vi "Offline_Analysis_SWSVM_newSelectionMethod_in_분석기_woF4.vi"(0 "LDA_matrix":path caption="LDA_matrix.txt", 1 "svm_model_file":string, 3 "Target_order.txt":path, 4 "mius_flash_order":path, 5 "Brain":path, 6 "Target":path, 7 "피험자이름":string="홍길동", 8 "Nontarget":path, 10 "DIscard Channel Info":i32[](array[numeric]), 11 "Save_path":string, 12 "in_matrix":path caption="in") -> ()   [LabVIEW 2014]
uses:
  <vilib>/Utility/file.llb/Read From Spreadsheet File (DBL).vi
  <vilib>/Analysis/Matrix/Numeric/Conversions/Array To Matrix - RA2.vi
  <vilib>/Analysis/Matrix/Numeric/Conversions/Array To Matrix - RA.vi
  <vilib>/Utility/file.llb/Read From Spreadsheet File (I64).vi
  <vilib>/Utility/file.llb/Write To Spreadsheet File (DBL).vi
  <vilib>/Utility/file.llb/Write To Spreadsheet File (I64).vi
  <vilib>/Utility/file.llb/Write To Spreadsheet File (string).vi
  <vilib>/Analysis/Matrix/NI_Matrix.lvlib
panel:
  out "ACC":i16
  out "Target_order":i64[](array[numeric])
  out "Selected_Target":i32[](array[numeric])
  out "Accuracy":i16[](array[numeric])
  out "error out":errorcluster
  in  "Random_num":i32=6
  in  "Flash_Repeat":i32=20
  in  "Frame_Length":i32=10
  in  "Sampling_Rate":dbl=250.0
  # "ERP_Parameter안씀. LDA바로 집어넣으면 됨"
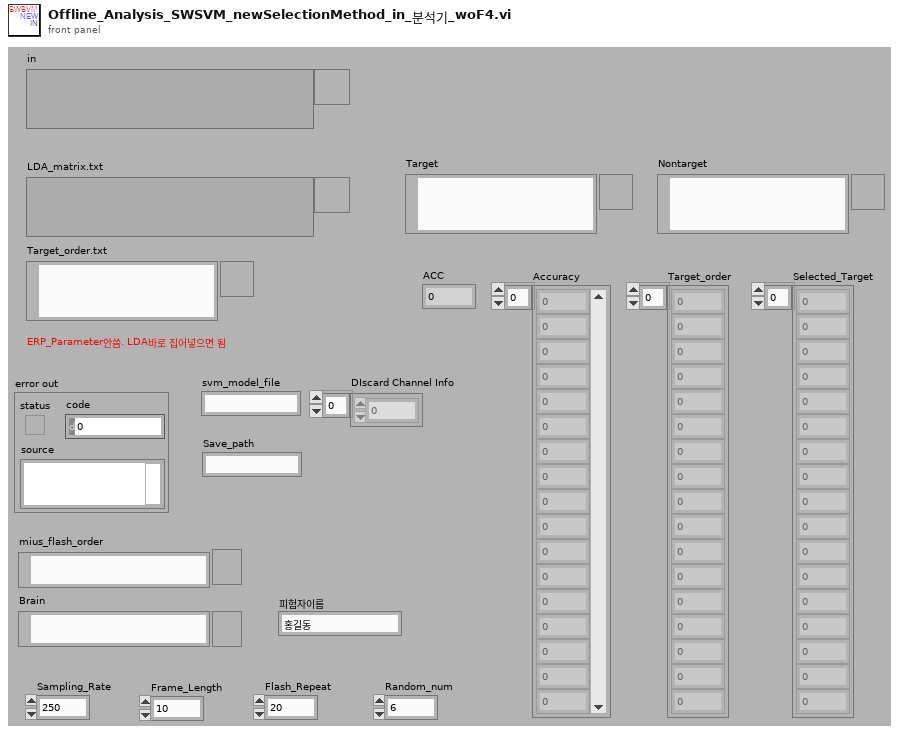
[diagram p1: front panel]
types:
  T1 = typedef "NI_Matrix.lvlib/RealMatrix.ctl" = dbl[][]
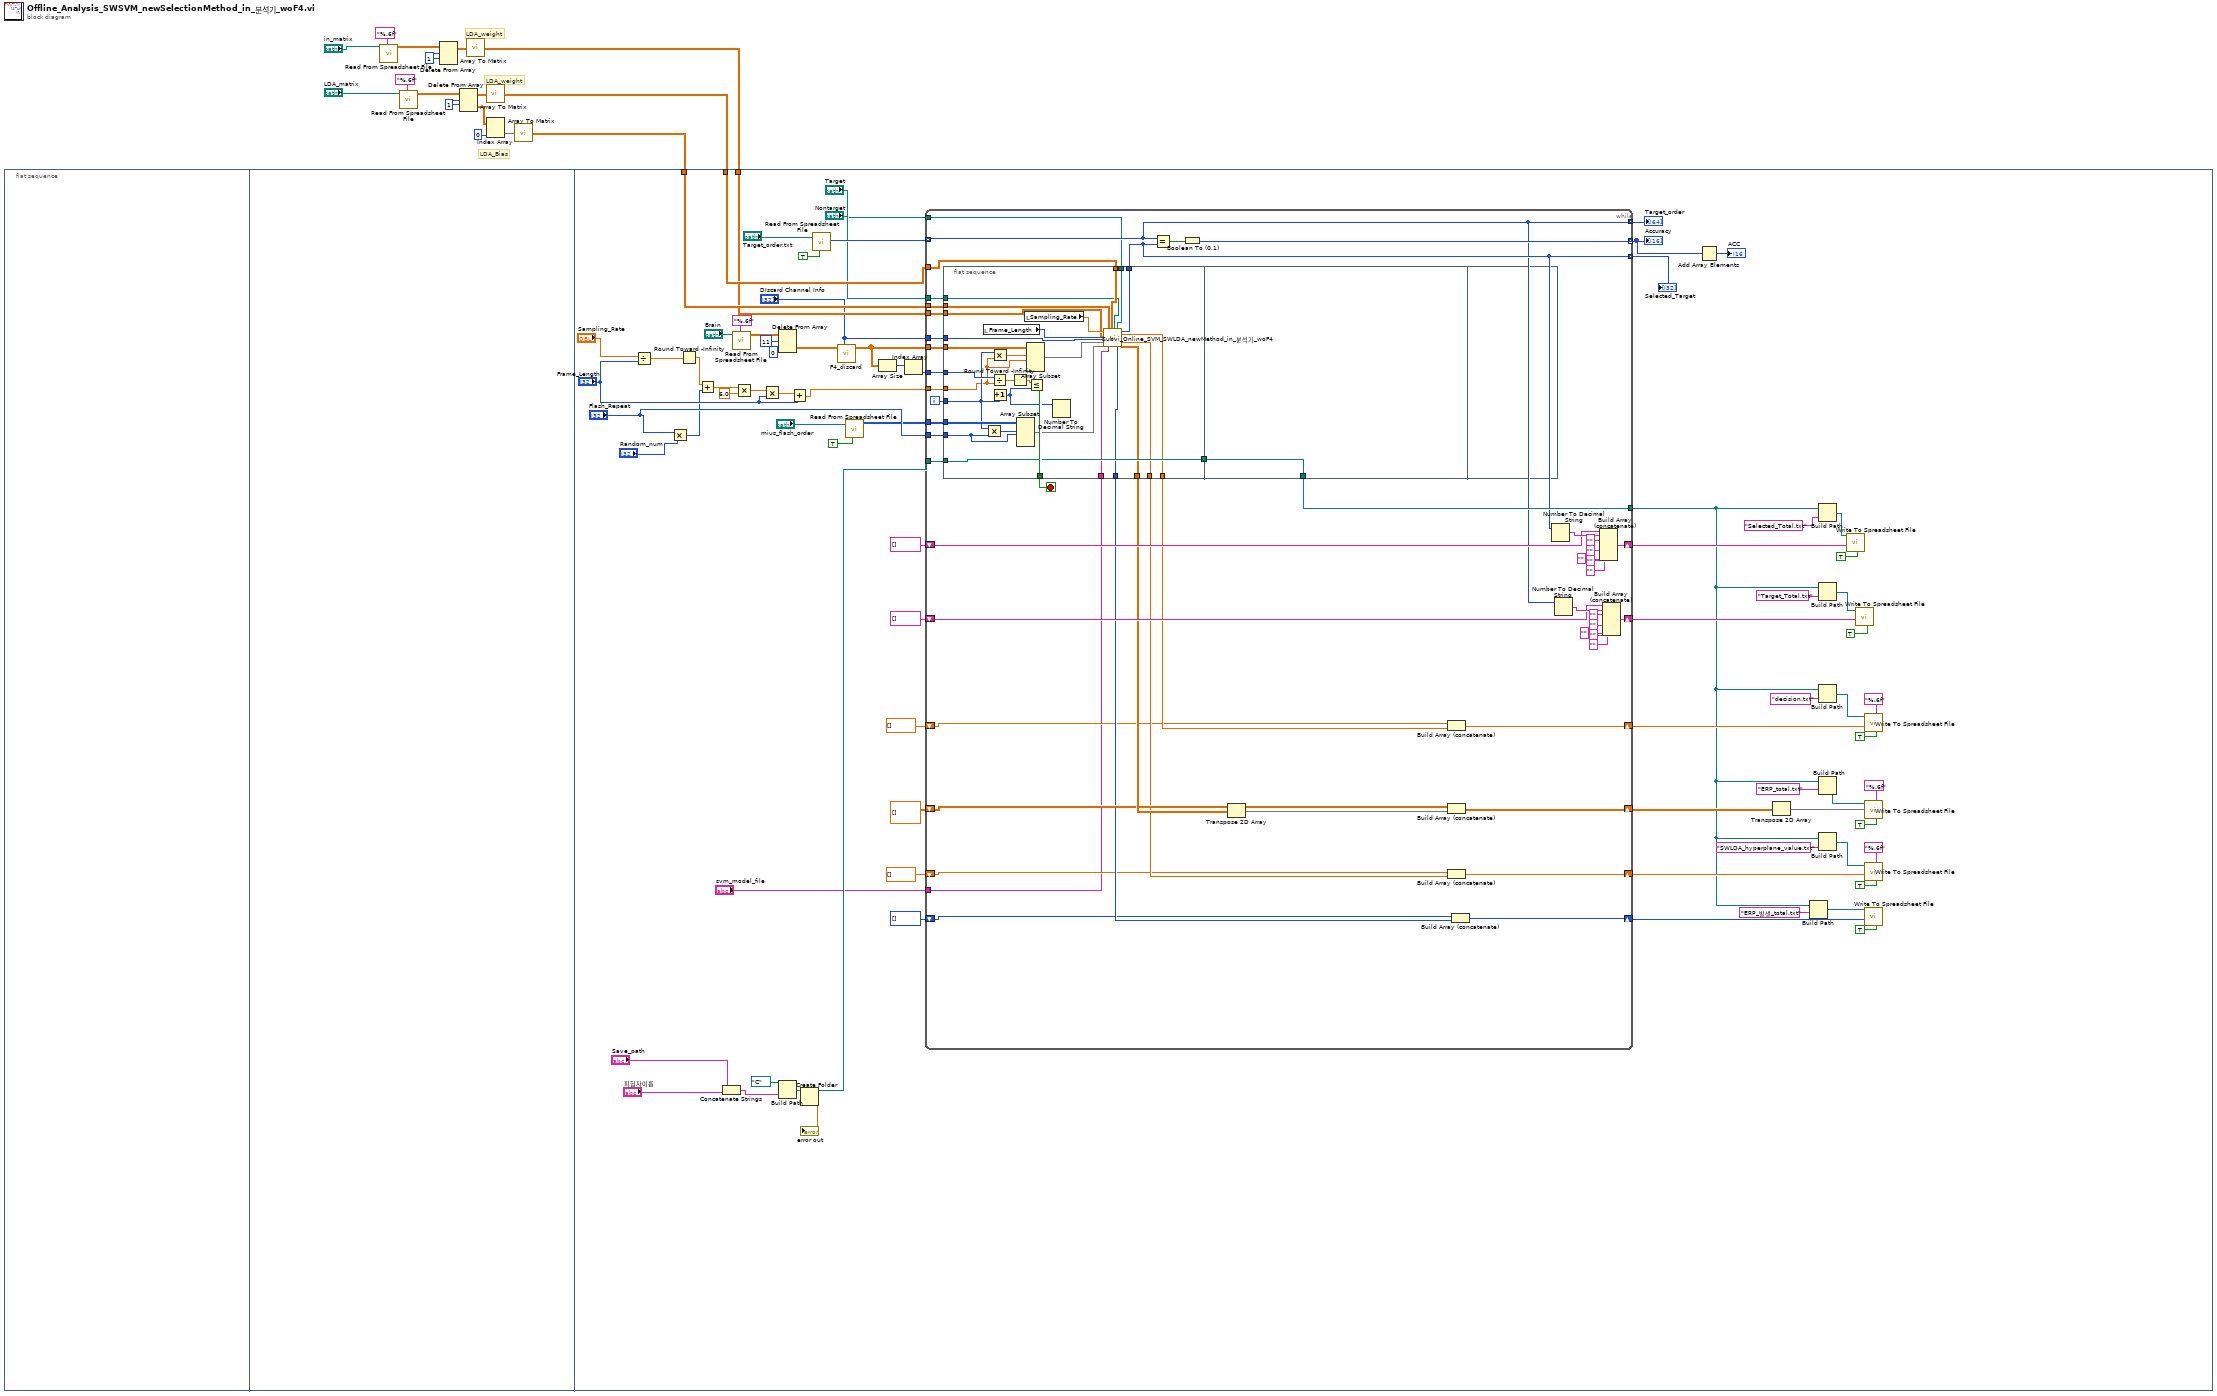
[diagram p0: block diagram]
diagram:
  w4 = 1 ("인덱스 (행)")
  w11 = 1 ("인덱스 (행)")
  # "LDA_weight"
  # "LDA_Bias"
  # "LDA_weight"
  n1 = flat-sequence {
    tunnel: w8 -> [w40]
    tunnel: w7 -> [w39]
    tunnel: w1 -> [w19]
    frame #0 {
    }
    frame #1 {
    }
    frame #2 {
      n2 = Divide(x="Sampling_Rate", y="Frame_Length") -> (x/y=w80:dbl)
      n3 = Multiply(x="Flash_Repeat", y="Random_num") -> (x*y=w83:i32)
      n4 = Round Toward -Infinity(1:w80) -> (0:w82:dbl)
      n5 = Add(x=w82, y=w83) -> (x+y=w85:dbl)
      n6 = Concatenate Strings("Save_path", "피험자이름") -> (w24:string)
      n7 = call-poly <vilib>:"Read From Spreadsheet File.vi"("format (%.3f)"="%.6f", "file path (dialog if empty)"="Brain") -> ("all rows"=w74:dbl[][])  [unwired: 5 in, 4 out]
      n8 = Multiply(x=w85, y=6.0) -> (x*y=w87:dbl)
      n9 = Multiply(x=w87, y="Frame_Length") -> (x*y=w89:dbl)
      n10 = Build Path(base path=path "C:/" ("path"), name or relative path=w24) -> (appended path=w92:path)
      n11 = Delete From Array(array=w74, length=11 ("길이"), index (col)=0 ("비활성화된 인덱스 (열)")) -> (deleted portion=w38:dbl[][])  [unwired: 1 in, 1 out]
      n12 = Add(x=w89, y="Frame_Length") -> (x+y=w90:dbl)
      n13 = Create Folder(path (use dialog)=w92) -> (created path=w94:path, error out=→"error out":errorcluster)  [unwired: 2 in, 1 out]
      n14 = call-poly <vilib>:"Read From Spreadsheet File.vi"("transpose (no:F)"=TRUE, "file path (dialog if empty)"="Target_order.txt") -> ("first row"=w68:i64[])  [unwired: 5 in, 4 out]
      n15 = call "F4_discard.vi"("DIscard Channel Info"="DIscard Channel Info", "Array"=w38) -> ("array w/ subset deleted"=w18:dbl[][])  [unwired: 9 in]
      n16 = call-poly <vilib>:"Read From Spreadsheet File.vi"("transpose (no:F)"=TRUE, "file path (dialog if empty)"="mius_flash_order") -> ("all rows"=w76:i64[][])  [unwired: 5 in, 4 out]
      n17 = Array Size(array=w18) -> (size(s)=w77:i32[])
      n18 = Index Array(array=w77) -> (element=w78:i32)  [unwired: 1 in]
      n19 = while {
        tunnel: w39 -> [w146]
        tunnel: w40 -> [w145]
        tunnel: w18 -> [w143]
        tunnel: w76 -> [w142]
        tunnel: w78 -> [w144]
        tunnel: w90 -> [w140]
        tunnel: "Flash_Repeat" -> [w141]
        tunnel: w94 -> [w139]
        tunnel: w68 -> [w117] mode=indexing
        tunnel: [w136] -> w60 mode=indexing
        tunnel: [w117] -> w65 mode=indexing
        tunnel: [w118] -> w66 mode=indexing
        tunnel: [w133] -> w26
        shift-right: [w120] -> w54
        shift-left: string[] [] -> [w119]
        shift-right: [w116] -> w53
        shift-left: string[] [] -> [w115]
        shift-right: [w112] -> w48
        shift-left: dbl[][] [] -> [w111]
        shift-right: [w109] -> w41
        shift-left: i16[] [] -> [w108]
        shift-right: [w106] -> w34
        shift-left: dbl[] [] -> [w105]
        shift-right: [w103] -> w27
        shift-left: dbl[] [] -> [w102]
        tunnel: "svm_model_file" -> [w101]
        tunnel: "Target" -> [w100]
        tunnel: "Nontarget" -> [w99]
        tunnel: w19 -> [w98]
        tunnel: "DIscard Channel Info" -> [w97]
        i -> [w135]
        stop <- w134 stop-if-true
        n20 = flat-sequence {
          tunnel: w146 -> [w175]
          tunnel: w145 -> [w174]
          tunnel: w144 -> [w173]
          tunnel: [w172] -> w134
          tunnel: w143 -> [w171]
          tunnel: w142 -> [w168]
          tunnel: w141 -> [w166]
          tunnel: w135 -> [w165]
          tunnel: w140 -> [w164]
          tunnel: w139 -> [w157]
          tunnel: [w157] -> w138
          tunnel: [w158] -> w118
          tunnel: [w156] -> w114
          tunnel: [w155] -> w110
          tunnel: [w153] -> w107
          tunnel: [w152] -> w104
          tunnel: w101 -> [w151]
          tunnel: w100 -> [w150]
          tunnel: w99 -> [w149]
          tunnel: w98 -> [w148]
          tunnel: w97 -> [w147]
          tunnel: w138 -> [w176]
          tunnel: [w176] -> w133
          frame #0 {
            n21 = local read "Frame_Length"() -> (w160:i32)
            n22 = Multiply(x=w165, y=w166) -> (x*y=w167:i32)
            n23 = Divide(x=w173, y=w164) -> (x/y=w163:dbl)
            n24 = Multiply(x=w165, y=w164) -> (x*y=w170:dbl)
            n25 = Increment(x=w165) -> (x+1=w159:i32)
            n26 = Round Toward -Infinity(1:w163) -> (0:w162:dbl)
            n27 = Array Subset(array=w168, index (row)=w167, length (row)=w166) -> (w154:i64[][])  [unwired: 2 in]
            n28 = local read "Sampling_Rate"() -> (w161:dbl)
            n29 = Array Subset(array=w171, index (row)=w170, length (row)=w164) -> (w169:dbl[][])  [unwired: 2 in]
            n30 = Less Or Equal?(x=w162, y=w159) -> (x <= y?=w172:bool)
            n31 = Number To Decimal String(number=w159) -> ()  [unwired: 1 in, 1 out]
            n32 = call "Subvi_Online_SVM_SWLDA_newMethod_in_분석기_woF4.vi"("rate"=w161, "samples per channel"=w160, "in"=w148, "DIscard Channel Info"=w147, "Brain_data_source"=w169, "Target_Flash_Order"=w154, "Value"=w175, "svm_model_file"=w151, "Matrix"=w174, "Target"=w150, "Nontarget"=w149) -> ("EPR_발생_total"=w155:i16[], "output-0~8"=w158:i32, "decision"=w152:dbl[], "SWLDA"=w153:dbl[], "ERP_Parameters"=w156:dbl[][])  [unwired: 4 in]
          }
          frame #1 {
          }
          frame #2 {
          }
        }
        n33 = Equal?(x=w117, y=w118) -> (x = y?=w137:bool)
        n34 = Boolean To (0,1)(Boolean=w137) -> (0, 1=w136:i16)
        n35 = Transpose 2D Array(2D array=w114) -> (transposed array=w113:dbl[][])
        n36 = Build Array (concatenate)(w102, w104) -> (w103:dbl[])
        n37 = Build Array (concatenate)(w111, w113) -> (w112:dbl[][])
        n38 = Build Array (concatenate)(w105, w107) -> (w106:dbl[])
        n39 = Build Array (concatenate)(w108, w110) -> (w109:i16[])
        n40 = Number To Decimal String(number=w118) -> (decimal integer string=w126:string)  [unwired: 1 in]
        n41 = Number To Decimal String(number=w117) -> (decimal integer string=w132:string)  [unwired: 1 in]
        n42 = Build Array (concatenate)(w119, w126, "" ("element"), "" ("element"), "" ("element"), "" ("element"), "" ("element")) -> (w120:string[])
        n43 = Build Array (concatenate)(w115, w132, "" ("element"), "" ("element"), "" ("element"), "" ("element"), "" ("element")) -> (w116:string[])
      }
      "Accuracy" <- w60
      "Selected_Target" <- w66
      "Target_order" <- w65
      n44 = Add Array Elements(numeric array=w60) -> (sum=→"ACC":i16)
      n45 = Transpose 2D Array(2D array=w48) -> (transposed array=w46:dbl[][])
      n46 = Build Path(base path=w26, name or relative path="ERP_발생_total.txt") -> (appended path=w43:path)
      n47 = Build Path(base path=w26, name or relative path="Selected_Total.txt") -> (appended path=w56:path)
      n48 = Build Path(base path=w26, name or relative path="Target_Total.txt") -> (appended path=w62:path)
      n49 = Build Path(base path=w26, name or relative path="decision.txt") -> (appended path=w28:path)
      n50 = Build Path(base path=w26, name or relative path="ERP_total.txt") -> (appended path=w49:path)
      n51 = Build Path(base path=w26, name or relative path="SWLDA_hyperplane_value.txt") -> (appended path=w36:path)
      n52 = call-poly <vilib>:"Write To Spreadsheet File.vi"("transpose? (no:F)"=TRUE, "1D data"=w54, "file path (dialog if empty)"=w56) -> ()  [unwired: 5 in, 1 out]
      n53 = call-poly <vilib>:"Write To Spreadsheet File.vi"("transpose? (no:F)"=TRUE, "1D data"=w53, "file path (dialog if empty)"=w62) -> ()  [unwired: 5 in, 1 out]
      n54 = call-poly <vilib>:"Write To Spreadsheet File.vi"("transpose? (no:F)"=TRUE, "format (%.3f)"="%.6f", "1D data"=w27, "file path (dialog if empty)"=w28) -> ()  [unwired: 4 in, 1 out]
      n55 = call-poly <vilib>:"Write To Spreadsheet File.vi"("transpose? (no:F)"=TRUE, "format (%.3f)"="%.6f", "2D data"=w46, "file path (dialog if empty)"=w49) -> ()  [unwired: 4 in, 1 out]
      n56 = call-poly <vilib>:"Write To Spreadsheet File.vi"("transpose? (no:F)"=TRUE, "format (%.3f)"="%.6f", "1D data"=w34, "file path (dialog if empty)"=w36) -> ()  [unwired: 4 in, 1 out]
      n57 = call-poly <vilib>:"Write To Spreadsheet File.vi"("transpose? (no:F)"=TRUE, "1D data"=w41, "file path (dialog if empty)"=w43) -> ()  [unwired: 5 in, 1 out]
    }
  }
  n58 = call-poly <vilib>:"Read From Spreadsheet File.vi"("format (%.3f)"="%.6f", "file path (dialog if empty)"="in_matrix") -> ("all rows"=w3:dbl[][])  [unwired: 5 in, 4 out]
  n59 = call-poly <vilib>:"Read From Spreadsheet File.vi"("format (%.3f)"="%.6f", "file path (dialog if empty)"="LDA_matrix") -> ("all rows"=w9:dbl[][])  [unwired: 5 in, 4 out]
  n60 = Delete From Array(array=w3, length=w4, index (row)=w4) -> (array with subset deleted=w5:dbl[][])  [unwired: 1 in, 1 out]
  n61 = Delete From Array(array=w9, length=w11, index (row)=w11) -> (deleted portion=w14:dbl[][], array with subset deleted=w13:dbl[][])  [unwired: 1 in]
  n62 = call-poly <vilib>:"Array To Matrix.vi"("Real 2D Array"=w5) -> ("Real Matrix"=w1:T1)
  n63 = call-poly <vilib>:"Array To Matrix.vi"("Real 2D Array"=w13) -> ("Real Matrix"=w8:T1)
  n64 = Index Array(array=w14, index (col)=0 ("인덱스")) -> (element=w12:dbl[])  [unwired: 1 in]
  n65 = call-poly <vilib>:"Array To Matrix.vi"("Real 1D Array"=w12) -> ("Real Matrix (Column Vector)"=w7:T1)
